vi "GDSString_FormatText.vi"(0 "TextIn":refnum<vi>, 5 "error in":errorcluster) -> (14 "TextOut":refnum<vi>, 19 "error out":errorcluster)   [LabVIEW 2020]
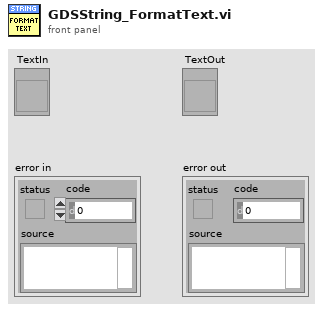
[diagram p1: front panel]
types:
  T1 = cluster{"Start":u32[], "Length":u32[], "Tag":string[]}
  T2 = enum16{"Bold", "Italic", "StrikOut", "UnderLine", "Color", "FontSize", "FontName"}
  T3 = cluster{"Style":enum16{"Bold", "Italic", "StrikOut", "UnderLine", "Color", "FontSize", "FontName"}, "Start":string, "End":string}[]
  T4 = cluster{"Text":string, "Formats":cluster{"Start":u32[], "Length":u32[], "Tag":string[]}[]}
  T5 = cluster{"Style":enum16{"Bold", "Italic", "StrikOut", "UnderLine", "Color", "FontSize", "FontName"}, "Start":string}[]
  T6 = cluster{"Start":u32[], "Length":u32[], "Tag":string[]}[]
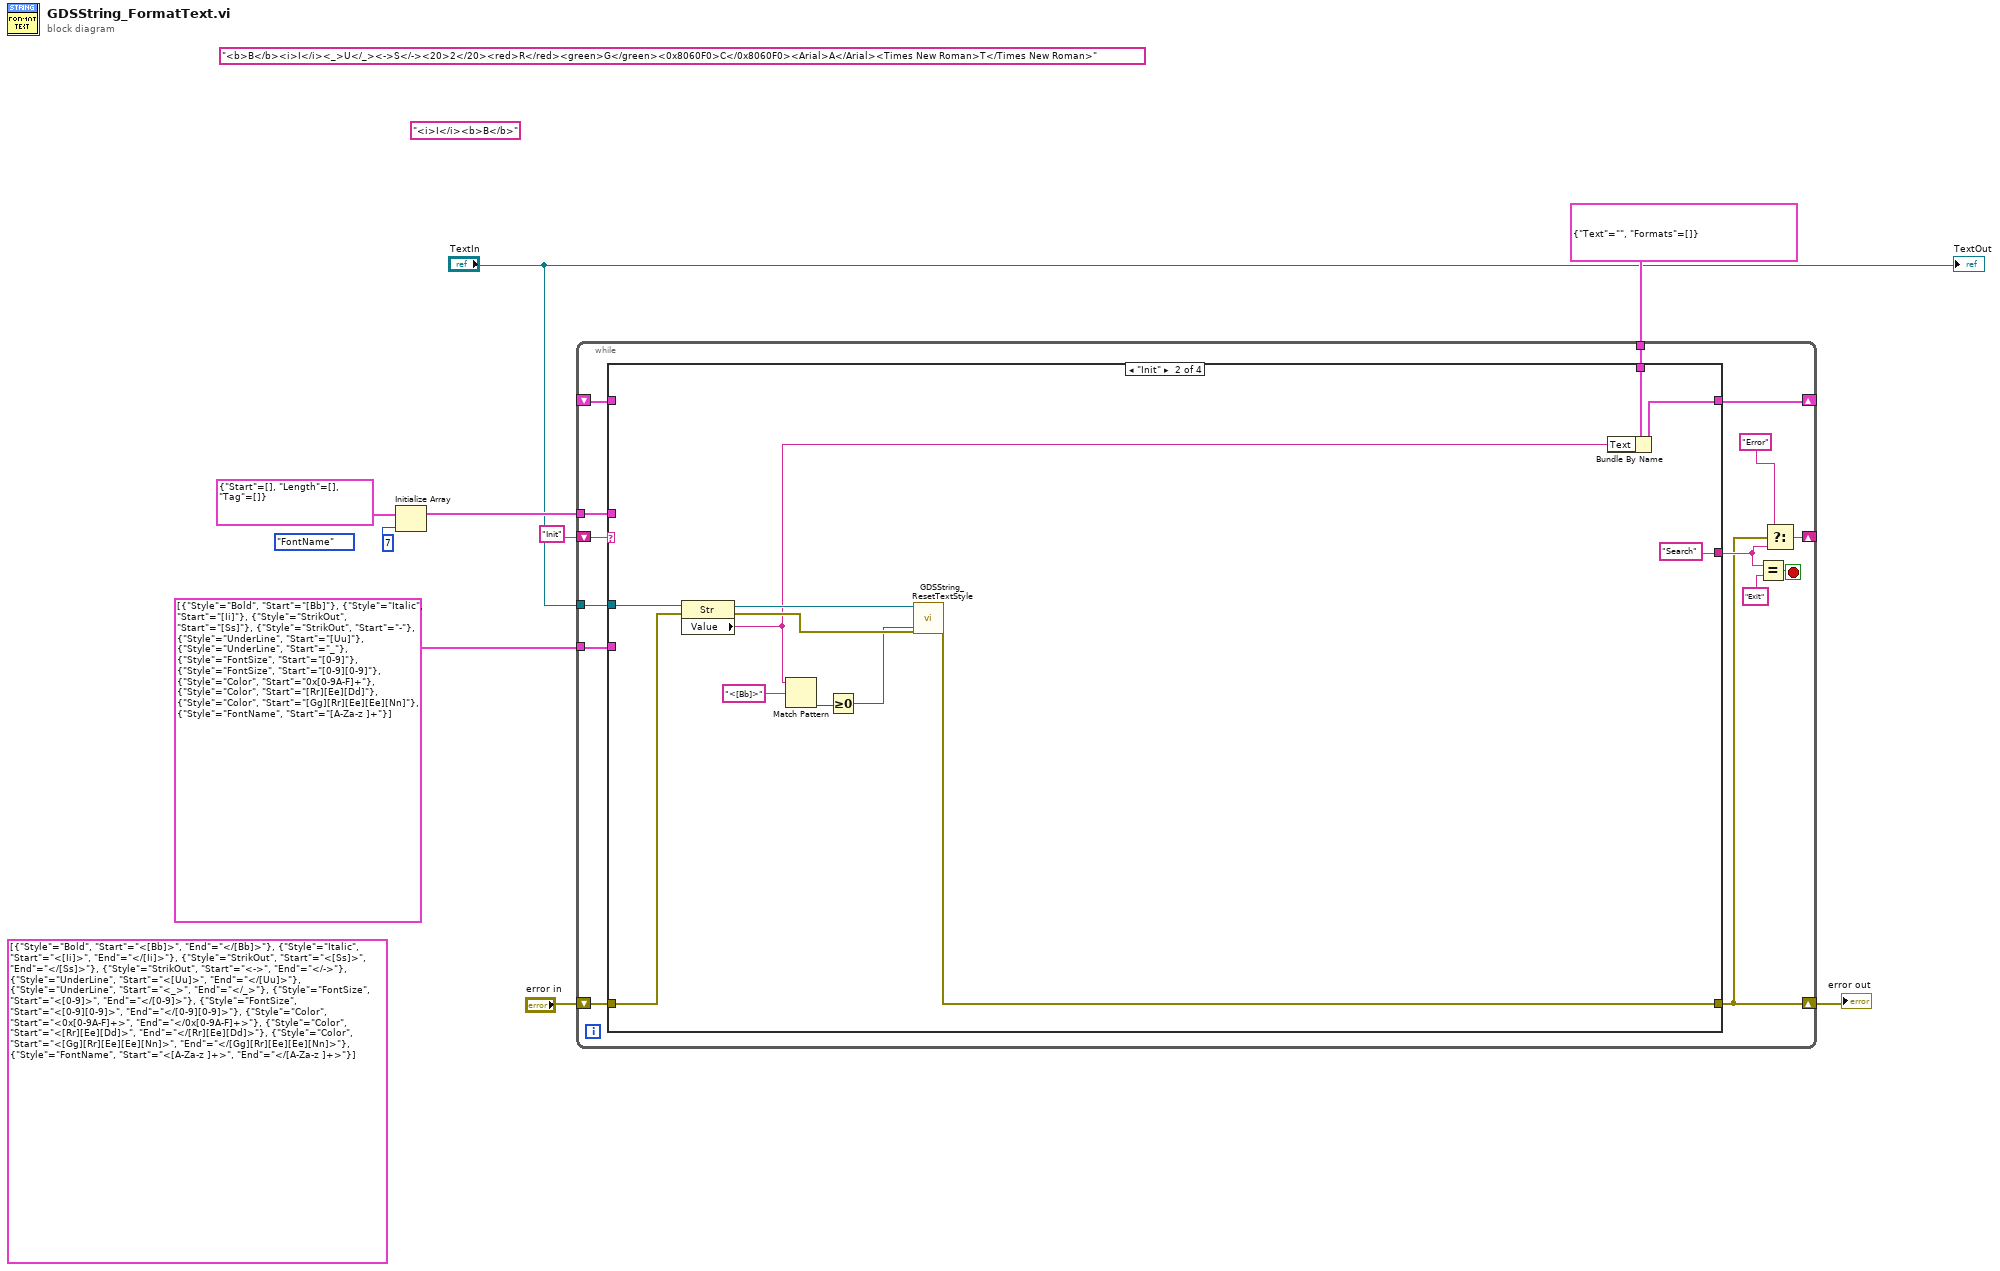
[diagram p0: block diagram]
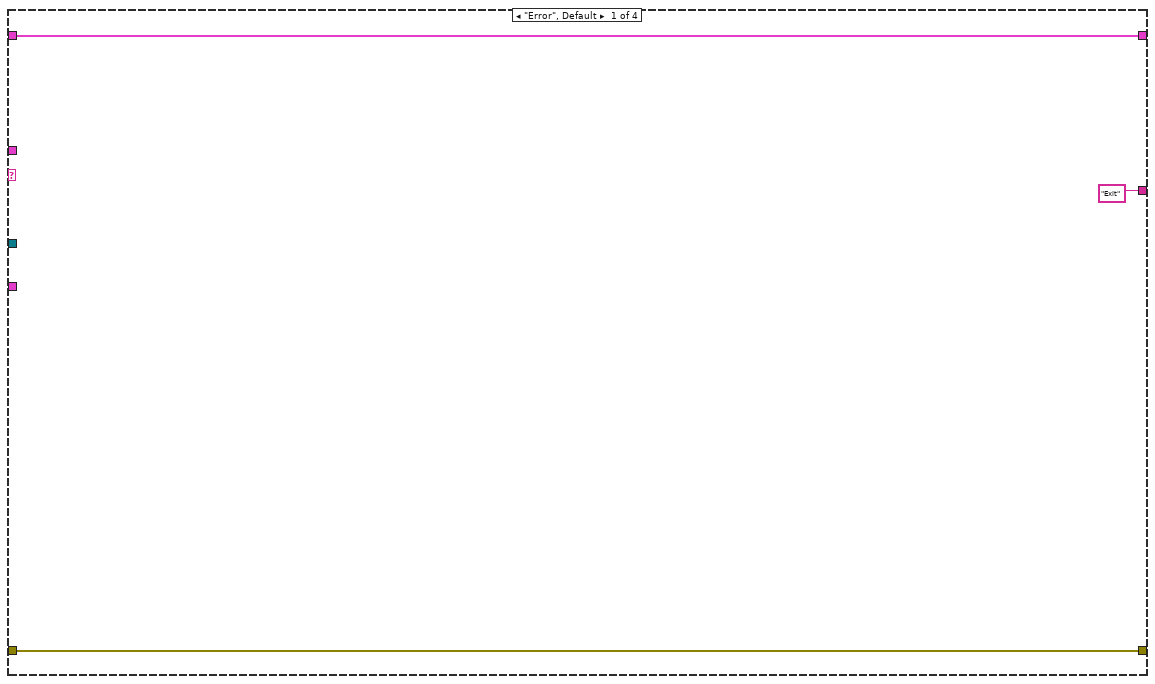
[diagram p2: hidden frame]
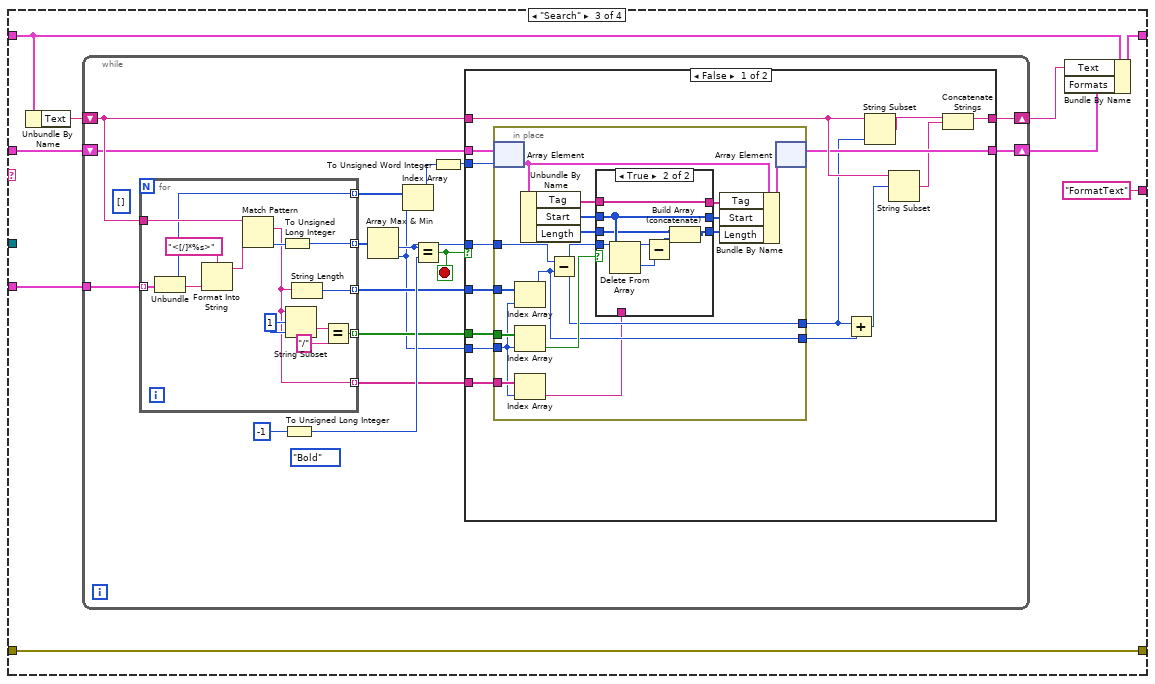
[diagram p3: hidden frame]
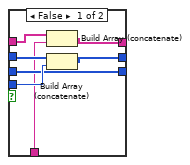
[diagram p4: hidden frame]
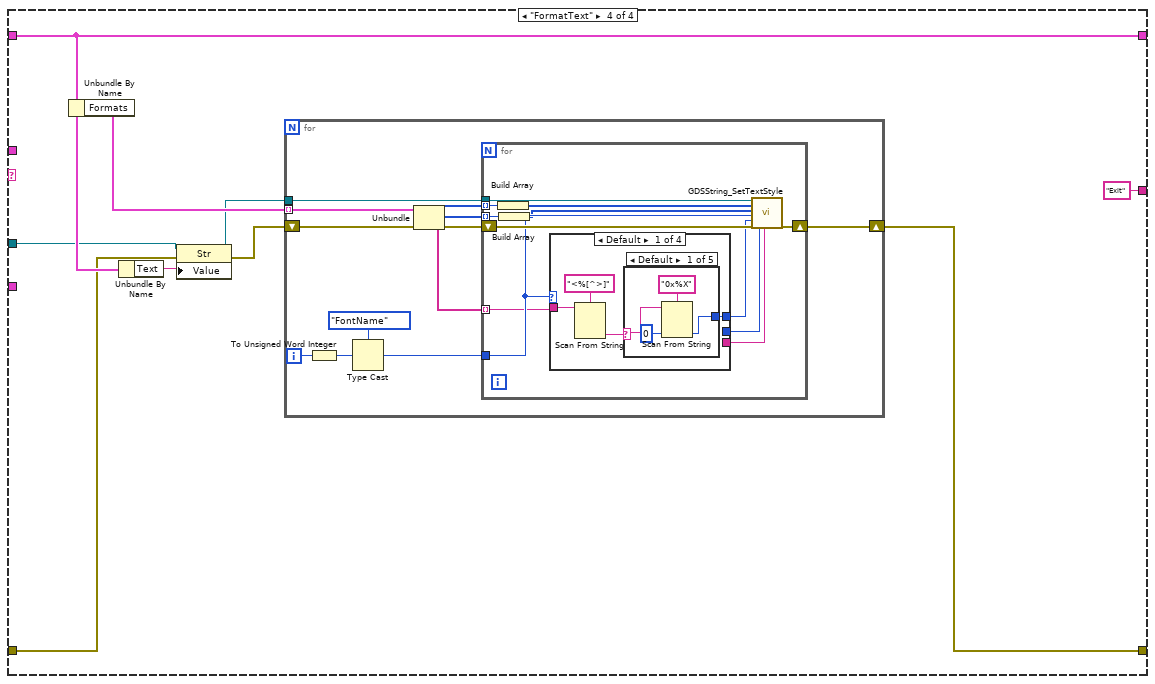
[diagram p6: hidden frame]
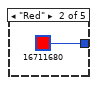
[diagram p7: hidden frame]
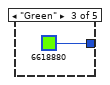
[diagram p8: hidden frame]
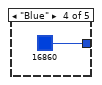
[diagram p9: hidden frame]
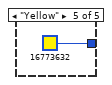
[diagram p10: hidden frame]
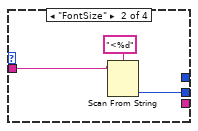
[diagram p11: hidden frame]
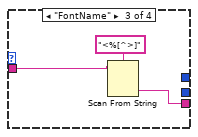
[diagram p12: hidden frame]
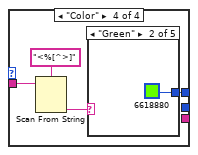
[diagram p13: hidden frame]
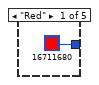
[diagram p14: hidden frame]
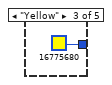
[diagram p15: hidden frame]
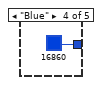
[diagram p16: hidden frame]
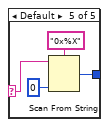
[diagram p17: hidden frame]
diagram:
  (unwired) T2."FontName" ("Style")
  (unwired) T3 [{"Style"=enum."Bold", "Start"="<[Bb]>", "End"="</[Bb]>"}, {"Style"=enum."Italic", "Start"="<[Ii]>", "End"="</[Ii]>"}, {"Style"=enum."StrikOut", "Start"="<[Ss]>", "End"="</[Ss]>"}, {"Style"=enum."StrikOut", "Start"="<->", "End"="</->"}, {"Style"=enum."UnderLine", "Start"="<[Uu]>", "End"="</[Uu]>"}, {"Style"=enum."UnderLine", "Start"="<_>", "End"="</_>"}, {"Style"=enum."FontSize", "Start"="<[0-9]>", "End"="</[0-9]>"}, {"Style"=enum."FontSize", "Start"="<[0-9][0-9]>", "End"="</[0-9][0-9]>"}, {"Style"=enum."Color", "Start"="<0x[0-9A-F]+>", "End"="</0x[0-9A-F]+>"}, {"Style"=enum."Color", "Start"="<[Rr][Ee][Dd]>", "End"="</[Rr][Ee][Dd]>"}, {"Style"=enum."Color", "Start"="<[Gg][Rr][Ee][Ee][Nn]>", "End"="</[Gg][Rr][Ee][Ee][Nn]>"}, {"Style"=enum."FontName", "Start"="<[A-Za-z ]+>", "End"="</[A-Za-z ]+>"}]
  (unwired) "<b>B</b><i>I</i><_>U</_><->S</-><20>2</20><red>R</red><green>G</green><0x8060F0>C</0x8060F0><Arial>A</Arial><Times New Roman>T</Times New Roman>" ("TextIn")
  (unwired) "<i>I</i><b>B</b>" ("TextIn")
  n1 = Initialize Array(T1 {"Start"=[], "Length"=[], "Tag"=[]}, 7 ("dimension size")) -> (w2:T6)
  n2 = while {
    shift-right: [w16] -> w7
    shift-left: "error in" -> [w23]
    shift-right: [w21] -> _
    shift-left: "Init" -> [w22]
    shift-right: [w15] -> _
    shift-left: _ -> [w14]
    tunnel: T4 {"Text"="", "Formats"=[]} -> [w13]
    tunnel: "TextIn" -> [w12]
    tunnel: T5 [{"Style"=enum."Bold", "Start"="[Bb]"}, {"Style"=enum."Italic", "Start"="[Ii]"}, {"Style"=enum."StrikOut", "Start"="[Ss]"}, {"Style"=enum."StrikOut", "Start"="-"}, {"Style"=enum."UnderLine", "Start"="[Uu]"}, {"Style"=enum."UnderLine", "Start"="_"}, {"Style"=enum."FontSize", "Start"="[0-9]"}, {"Style"=enum."FontSize", "Start"="[0-9][0-9]"}, {"Style"=enum."Color", "Start"="0x[0-9A-F]+"}, {"Style"=enum."Color", "Start"="[Rr][Ee][Dd]"}, {"Style"=enum."Color", "Start"="[Gg][Rr][Ee][Ee][Nn]"}, {"Style"=enum."FontName", "Start"="[A-Za-z ]+"}] -> [w11]
    tunnel: w2 -> [w10]
    stop <- w20 stop-if-true
    n3 = case shown="\"Init\"" w22 {
      tunnel: w23 -> [w26 w32 w46 w130]
      tunnel: [w26 w31 w46 w134] -> w16
      tunnel: ["Exit" "Search" "FormatText" "Exit"] -> w17
      tunnel: [w24 w37 w39 w131] -> w15
      tunnel: w14 -> [w24 _ w41 w131]
      tunnel: w13 -> [_ w36 _ _]
      tunnel: w12 -> [_ w35 _ w128]
      tunnel: w11 -> [_ _ w44 _]
      tunnel: w10 -> [_ _ w43 _]
      frame "Error", Default {
      }
      frame "Init" {
        n4 = property class="Str"(reference=w35, error in=w32) -> (reference out=w34:refnum<vi>, error out=w33:errorcluster, "Value"=w30:string)
        n5 = Match Pattern(string=w30, regular expression="<[Bb]>" ("Start")) -> (offset past match=w28:i32)  [unwired: 4 out]
        n6 = Greater Or Equal To 0?(x=w28) -> (x >= 0?=w27:bool)
        n7 = call "GDSString_ResetTextStyle.vi"("TextIn"=w34, "ResetBold(True)"=w27, "error in"=w33) -> ("error out"=w31:errorcluster)  [unwired: 15 in, 1 out]
        n8 = Bundle By Name(cluster=w36, "Text"=w30) -> (w37:T4)
      }
      frame "Search" {
        n9 = Unbundle By Name(w41) -> ("Text"=w45:string)
        n10 = while {
          shift-right: [w60] -> w42
          shift-left: w45 -> [w61]
          tunnel: w44 -> [w64]
          shift-right: [w53] -> w40
          shift-left: w43 -> [w58]
          stop <- w59 stop-if-true
          (unwired) T2."Bold" ("Style")
          (unwired) u32[] []
          n11 = for {
            tunnel: w61 -> [w124]
            tunnel: w64 -> [w126] mode=indexing
            tunnel: [w118] -> w57 mode=indexing
            tunnel: [w117] -> w56 mode=indexing
            tunnel: [w116] -> w55 mode=indexing
            tunnel: [w114] -> w52 mode=indexing
            tunnel: [w113] -> w48 mode=indexing
            w115 = 1 ("offset (0)")
            n12 = Unbundle(w126) -> ("Style"=w114:T2, "Start"=w122:string)
            n13 = Format Into String(format string="<[/]*%s>", w122) -> (resulting string=w121:string)  [unwired: 2 in, 1 out]
            n14 = Match Pattern(string=w124, regular expression=w121) -> (match substring=w113:string, offset past match=w125:i32)  [unwired: 3 out]
            n15 = To Unsigned Long Integer(number=w125) -> (unsigned 32bit integer=w117:u32)
            n16 = String Subset(string=w113, offset (0)=w115, length (rest)=w115) -> (substring=w120:string)
            n17 = String Length(string=w113) -> (length=w116:i32)
            n18 = Equal?(x=w120, y="/") -> (x = y?=w118:bool)
          }
          n19 = To Unsigned Long Integer(number=-1) -> (unsigned 32bit integer=w62:u32)
          n20 = Array Max & Min(array=w56) -> (min value=w54:u32, min index (indices)=w49:i32)  [unwired: 2 out]
          n21 = Index Array(array=w52, index=w49) -> (element=w51:T2)
          n22 = Equal?(x=w54, y=w62) -> (x = y?=w59:bool)
          n23 = To Unsigned Word Integer(number=w51) -> (unsigned 16bit integer=w50:u16)
          n24 = case shown="False" w59 {
            tunnel: w61 -> [w73 w112]
            tunnel: [w75 w112] -> w60
            tunnel: w58 -> [w79 w111]
            tunnel: w50 -> [w77 _]
            tunnel: w57 -> [w78 _]
            tunnel: w55 -> [w76 _]
            tunnel: w54 -> [w74 _]
            tunnel: [w72 w111] -> w53
            tunnel: w49 -> [w66 _]
            tunnel: w48 -> [w65 _]
            frame False {
              n25 = in-place {
                in-place-border: w78 -> [w96]
                in-place-border: w66 -> [w80]
                in-place-border: w76 -> [w92]
                in-place-border: w74 -> [w88]
                in-place-border: [w86] -> w70
                in-place-border: [w85] -> w69
                in-place-border: w65 -> [w84]
                n26 = in-place-array #1(w79, w77) -> (w91:T1)
                n27 = Index Array(array=w92, index=w80) -> (element=w85:i32)
                n28 = Index Array(array=w96, index=w80) -> (element=w95:bool)
                n29 = Index Array(array=w84, index=w80) -> (element=w82:string)
                n30 = Unbundle By Name(w91) -> ("Tag"=w83:string[], "Start"=w94:u32[], "Length"=w93:u32[])
                n31 = Subtract(x=w88, y=w85) -> (x-y=w86:u32)
                n32 = case shown="True" w95 {
                  tunnel: w94 -> [w103 w110]
                  tunnel: w93 -> [w100 w107]
                  tunnel: [w102 w110] -> w90
                  tunnel: w86 -> [w101 w109]
                  tunnel: [w100 w105] -> w89
                  tunnel: w83 -> [w99 w104]
                  tunnel: w82 -> [w98 _]
                  tunnel: [w97 w104] -> w81
                  frame False {
                    n33 = Build Array (concatenate)(w99, w98) -> (w97:string[])
                    n34 = Build Array (concatenate)(w103, w101) -> (w102:u32[])
                  }
                  frame True {
                    n35 = Delete From Array(array=w110) -> (deleted portion=w108:u32)  [unwired: 2 in, 1 out]
                    n36 = Subtract(x=w109, y=w108) -> (x-y=w106:u32)
                    n37 = Build Array (concatenate)(w107, w106) -> (w105:u32[])
                  }
                }
                n38 = Bundle By Name(cluster=w91, "Tag"=w81, "Start"=w90, "Length"=w89) -> (w87:T1)
                n39 = in-place-array #1(w87) -> (w72:T6)  [unwired: 1 out]
              }
              n40 = Add(x=w70, y=w69) -> (x+y=w68:u32)
              n41 = String Subset(string=w73, length (rest)=w70) -> (substring=w71:string)  [unwired: 1 out]
              n42 = String Subset(string=w73, offset (0)=w68) -> (substring=w67:string)  [unwired: 1 out]
              n43 = Concatenate Strings(w71, w67) -> (w75:string)
            }
            frame True {
            }
          }
        }
        n44 = Bundle By Name(cluster=w41, "Text"=w42, "Formats"=w40) -> (w39:T4)
      }
      frame "FormatText" {
        n45 = Unbundle By Name(w131) -> ("Formats"=w135:T6)
        n46 = Unbundle By Name(w131) -> ("Text"=w132:string)
        n47 = property class="Str"(reference=w128, error in=w130, "Value"=w132) -> (reference out=w127:refnum<vi>, error out=w129:errorcluster)
        n48 = for {
          tunnel: w127 -> [w146]
          tunnel: w135 -> [w144] mode=indexing
          shift-right: [w137] -> w134
          shift-left: w129 -> [w145]
          i -> [w140]
          n49 = To Unsigned Word Integer(number=w140) -> (unsigned 16bit integer=w139:u16)
          n50 = Type Cast(type=T2."FontName" ("Style"), x=w139) -> (*(type *) &x=w138:T2)
          n51 = Unbundle(w144) -> ("Start"=w143:u32[], "Length"=w142:u32[], "Tag"=w136:string[])
          n52 = for {
            tunnel: w146 -> [w158]
            tunnel: w143 -> [w156] mode=indexing
            tunnel: w142 -> [w155] mode=indexing
            tunnel: w138 -> [w151]
            shift-right: [w148] -> w137
            shift-left: w145 -> [w157]
            tunnel: w136 -> [w147] mode=indexing
            n53 = Build Array(w156) -> (w150:u32[])
            n54 = Build Array(w155) -> (w149:u32[])
            n55 = case shown="Default" w151 {
              tunnel: w147 -> [w162 w173 w176 w179]
              tunnel: [_ w171 _ _] -> w154
              tunnel: [_ _ w174 _] -> w153
              tunnel: [w159 _ _ w177] -> w152
              frame Default {
                n56 = Scan From String(format string="<%[^>]", input string=w162) -> (output 1=w160:string)  [unwired: 2 in, 4 out]
                n57 = case shown="Default" w160 {
                  selector: w160 -> [w166 _ _ _ _]
                  tunnel: [w163 u32 16711680 u32 6618880 u32 16860 u32 16773632] -> w159
                  frame Default {
                    n58 = Scan From String(format string="0x%X", input string=w166, default 1=u32 0 ("default value 1")) -> (output 1=w163:u32)  [unwired: 2 in, 3 out]
                  }
                  frame "Red" {
                  }
                  frame "Green" {
                  }
                  frame "Blue" {
                  }
                  frame "Yellow" {
                  }
                }
              }
              frame "FontSize" {
                n59 = Scan From String(format string="<%d", input string=w173) -> (output 1=w171:i32)  [unwired: 2 in, 4 out]
              }
              frame "FontName" {
                n60 = Scan From String(format string="<%[^>]", input string=w176) -> (output 1=w174:string)  [unwired: 2 in, 4 out]
              }
              frame "Color" {
                n61 = Scan From String(format string="<%[^>]", input string=w179) -> (output 1=w178:string)  [unwired: 2 in, 4 out]
                n62 = case shown="\"Green\"" w178 {
                  selector: w178 -> [_ _ _ _ w188]
                  tunnel: [u32 16711680 u32 6618880 u32 16775680 u32 16860 w186] -> w177
                  frame "Red" {
                  }
                  frame "Green" {
                  }
                  frame "Yellow" {
                  }
                  frame "Blue" {
                  }
                  frame Default {
                    n63 = Scan From String(format string="0x%X", input string=w188, default 1=u32 0 ("default value 1")) -> (output 1=w186:u32)  [unwired: 2 in, 3 out]
                  }
                }
              }
            }
            n64 = call "GDSString_SetTextStyle.vi"("TextIn"=w158, "Start"=w150, "Length"=w149, "Style"=w151, "Color"=w152, "error in"=w157, "Size"=w154, "FontName"=w153) -> ("error out"=w148:errorcluster)  [unwired: 10 in, 1 out]
          }
        }
      }
    }
    n65 = Equal?(x=w17, y="Exit") -> (x = y?=w20:bool)
    n66 = Select(t="Error", s=w16, f=w17) -> (s? t:f=w21:string)
  }
  "error out" <- w7
  "TextOut" <- "TextIn"
